vi "Post-Launch Initialize.vi"(7 "GUI Reference":refnum<vi>, 8 "error in (no error)":errorcluster, 11 "Engine in":refnum<class "Engine.lvclass">) -> (0 "error out":errorcluster, 3 "Engine out":refnum<class "Engine.lvclass">, 4 "Registered Events":T1, 6 "Self Enqueuer":refnum<class "Message Enqueuer.lvclass">)   [LabVIEW 2023, in "Engine.lvlib" / "Engine.lvclass"]
doc: "<b>Post-Launch Initialize</b>\nThis routine performs all of the necessary steps prior to entering the actor state engine.\n\nAncestor classes can override the following routines called in this routine:\n1. <b>Link Control References</b> - Stores GUI control references to class private data\n2. <b>Pre-Actor</b> - Performs any relevant steps after the references are stored in class private data\n3. <b>Post-Register</b> - Performs any necessary actions immediately prior to entering the class state machine.\n\nSpecial Inputs:\n<b>GUI Reference</b> calling VI reference - this expects the actor core VI reference\n\nReturns:\n<b>Self Enqueuer</b> Message Queue for the calling actor, the means to send self addressed messages\n<b>Registered Events</b> This should be wired to dynamic events terminal in the actor's state machine."
uses:
  Library/Engine.lvclass
  builds/Framework/Actor Framework.lvlibp/1abvi3w/vi.lib/ActorFramework/Message Enqueuer/Message Enqueuer.lvclass
  builds/Framework/Panel Manager.lvlibp/Panel/Panel Helper/Panel Events.ctl
  builds/Framework/Panel Manager.lvlibp/Panel/Panel Helper/Events.ctl
  Custom Controls/Events.ctl
  Custom Controls/SystemEvents.ctl
  Custom Controls/Faults.ctl
  Custom Controls/Status.ctl
  Custom Controls/OtherEvents.ctl
  Custom Controls/AbstractMessage.ctl
  Library/Engine.lvclass/Engine.ctl
  Accessors/Write VI Ref.vi
  Accessors/Read Events.vi
  builds/Framework/Panel Manager.lvlibp/Library/Panel Actor.lvclass
  builds/Framework/Panel Manager.lvlibp/Panel/Panel Helper/Panel Helper.lvclass
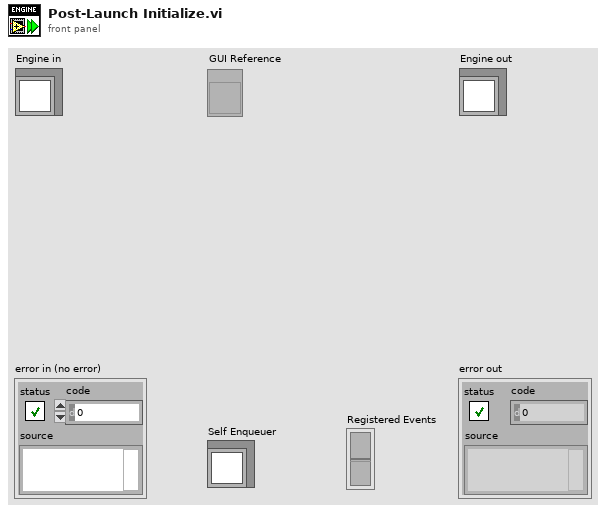
[diagram p1: front panel]
types:
  T1 = cluster{"Pnl Actor":refnum<event-registration>, "Event Registration Refnum":refnum<event-registration>}
  T2 = typedef "Engine.lvlib/Engine.lvclass/Events.ctl" = cluster{"System":T3, "Other":T4}
  T3 = typedef "Engine.lvlib/Engine.lvclass/SystemEvents.ctl" = cluster{"Fault Monitor":refnum<user-event>, "Status":refnum<user-event>}
  T4 = typedef "Engine.lvlib/Engine.lvclass/OtherEvents.ctl" = cluster{"Launch":refnum<user-event>, "AbstractMessage":refnum<user-event>}
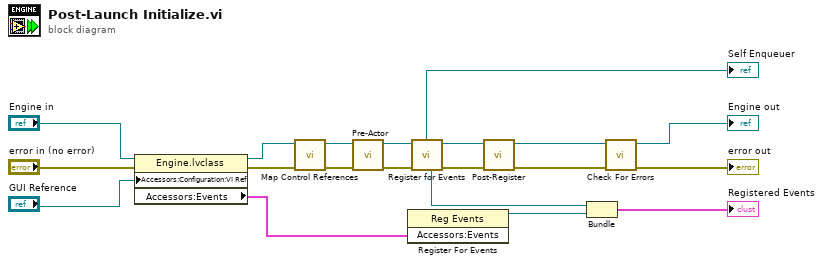
[diagram p0: block diagram]
diagram:
  n1 = property class="Engine.lvclass"(reference="Engine in", error in="error in (no error)", "Accessors:Configuration:VI Ref"="GUI Reference") -> (reference out=w4:refnum<class "Engine.lvclass">, error out=w3:errorcluster, "Accessors:Events"=w13:T2)
  n2 = call "Map Control References.vi"("error in (no error)"=w3, "Engine in"=w4) -> ("error out"=w1:errorcluster, "Engine out"=w2:refnum<class "Engine.lvclass">)  [unwired: 8 in]
  n3 = call-dynamic "Pre-Actor.vi"("error in (no error)"=w1, "Engine in"=w2) -> ("error out"=w15:errorcluster, "Engine out"=w16:refnum<class "Engine.lvclass">)  [unwired: 8 in]
  n4 = register-events(w13) -> (reference out=w12:refnum<event-registration>)  [unwired: 2 in, 1 out]
  n5 = call "Register for Events.vi"("Error In"=w15, "Panel Actor in"=w16) -> ("Error Out"=w20:errorcluster, "Panel Actor out"=w19:refnum<class "Engine.lvclass">, "Pnl Actor"=w11:refnum<event-registration>, "Self Enqueuer"=→"Self Enqueuer":refnum<class "Message Enqueuer.lvclass">)  [unwired: 6 in]
  n6 = call-dynamic "Post-Register.vi"("error in (no error)"=w20, "Engine in"=w19) -> ("error out"=w18:errorcluster, "Engine out"=w7:refnum<class "Engine.lvclass">)  [unwired: 8 in]
  n7 = Bundle("Pnl Actor"=w11, "Event Registration Refnum"=w12) -> (→"Registered Events":T1)  [unwired: 1 in]
  n8 = call "Check For Errors.vi"("error in"=w18, "Engine in"=w7) -> ("error out"=→"error out":errorcluster, "Engine out"=→"Engine out":refnum<class "Engine.lvclass">)  [unwired: 8 in]
